vi "reprTextual.vi"(8 "error in (no error)":errorcluster, 11 "RoundBuoy in":refnum<class "RoundBuoy.lvclass">) -> (0 "error out":errorcluster, 2 "Description":string, 3 "RoundBuoy out":refnum<class "RoundBuoy.lvclass">)   [LabVIEW 2011, in "RoundBuoy.lvclass"]
uses:
  RoundBuoy.lvclass
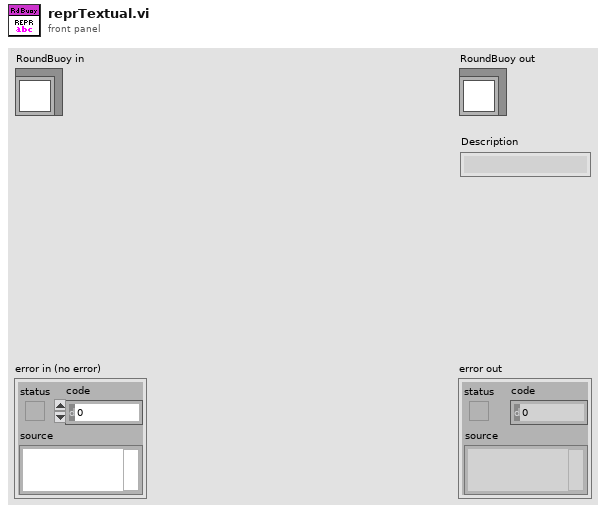
[diagram p1: front panel]
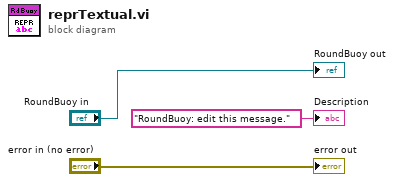
[diagram p0: block diagram]
diagram:
  "error out" <- "error in (no error)"
  "RoundBuoy out" <- "RoundBuoy in"
  "Description" <- "RoundBuoy: edit this message." ("Description")
